vi "sendValue.vi"(8 "error in (no error)":errorcluster, 10 "data":variant, 11 "settingsAppliedDomeController in":refnum<class "settingsAppliedDomeController.lvclass">) -> (0 "error out":errorcluster, 2 "function return":i32, 3 "settingsAppliedDomeController out":refnum<class "settingsAppliedDomeController.lvclass">)   [LabVIEW 2016, in "SALLV_AtDome_Messaging.lvlib" / "settingsAppliedDomeController.lvclass"]
uses:
  settingsAppliedDomeController.lvclass
  ts_sallv_AtDome/DataTypes/logevent_settingsAppliedDomeController.ctl
  ts_sallv_AtDome/SALLV_AtDome.lvlib
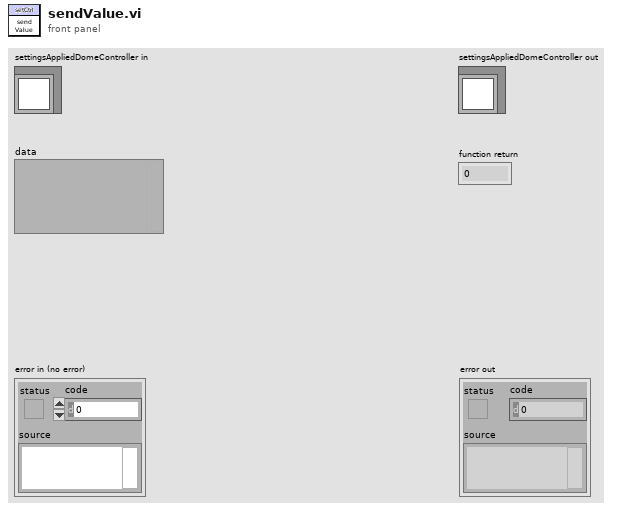
[diagram p1: front panel]
types:
  T1 = typedef "SALLV_AtDome.lvlib/logevent_settingsAppliedDomeController.ctl" = cluster{"rainSensorActivated":bool, "cloudSensorActivated":bool, "tolerance":sgl, "highSpeedDistance":sgl, "learnManual":i32, "watchdogTimer":sgl, "reversalDelay":sgl, "autoShutdownActivated":bool, "priority":i32}
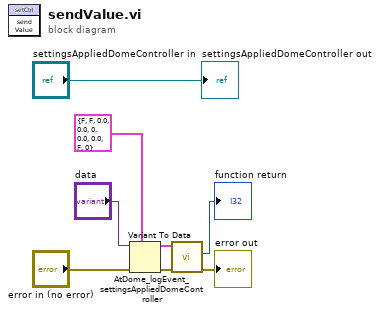
[diagram p0: block diagram]
diagram:
  n1 = Variant To Data(error in="error in (no error)", type=T1 {"rainSensorActivated"=FALSE, "cloudSensorActivated"=FALSE, "tolerance"=0.0, "highSpeedDistance"=0.0, "learnManual"=0, "watchdogTimer"=0.0, "reversalDelay"=0.0, "autoShutdownActivated"=FALSE, "priority"=0} ("logevent_settingsAppliedDomeController_Ctl"), Variant="data") -> (data=w2:T1, error out=w3:errorcluster)
  n2 = call "AtDome_logEvent_settingsAppliedDomeController.vi"("error in (no error)"=w3, "logevent_settingsAppliedDomeController_Ctl"=w2) -> ("error out"=→"error out":errorcluster, "function return"=→"function return":i32)  [unwired: 7 in, 1 out]
  "settingsAppliedDomeController out" <- "settingsAppliedDomeController in"
